vi "DataXML addNode.vi"(6 "allow repeat? (F)":bool, 7 "add_root? (F)":bool, 8 "error in (no error)":errorcluster, 9 "add tag name":string, 10 "parent node":refnum<k20>, 11 "DataXML in":refnum<class "DataXML.lvclass">) -> (0 "error out":errorcluster, 2 "new element":refnum<k20>, 3 "DataXML out":refnum<class "DataXML.lvclass">)   [LabVIEW 2018, in "DataXML.lvclass"]
uses:
  DataXML.lvclass
  DataXML.lvclass/DataXML.ctl
  <resource>/objmgr/DOMUserDefRef.rc
  <vilib>/xml/NI_XML.lvlib
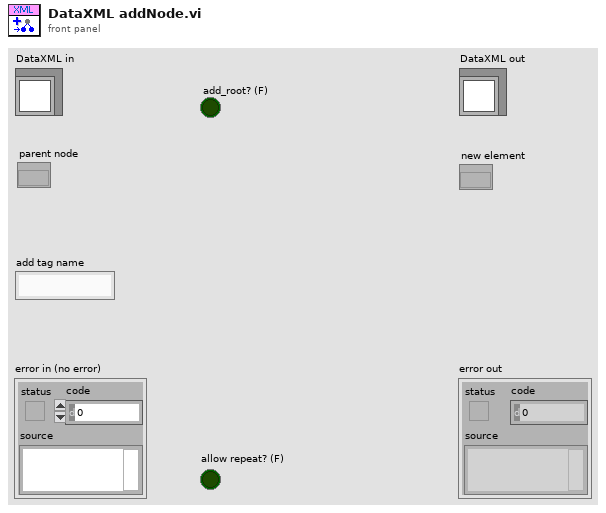
[diagram p1: front panel]
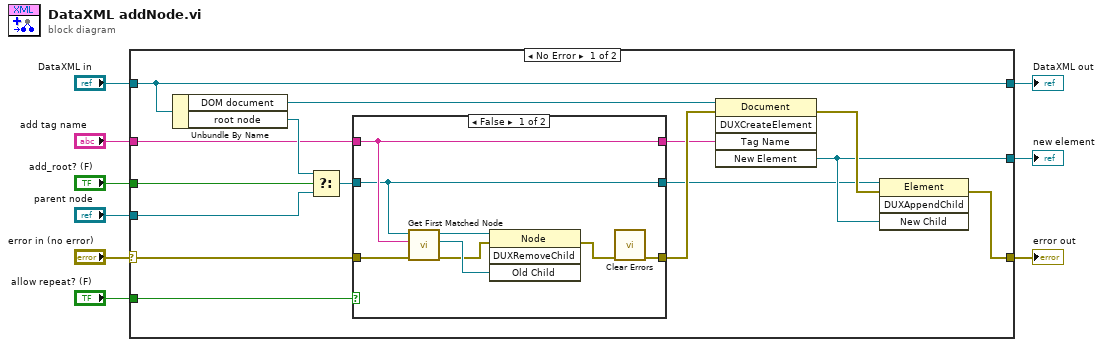
[diagram p0: block diagram]
diagram:
  n1 = case shown="No Error" "error in (no error)" {
    selector: "error in (no error)" -> [w15 w37]
    tunnel: [w18 w37] -> w8
    tunnel: [w24 w36] -> w6
    tunnel: "DataXML in" -> [w24 w36]
    tunnel: "parent node" -> [w21 _]
    tunnel: "add tag name" -> [w16 _]
    tunnel: "add_root? (F)" -> [w20 _]
    tunnel: [w17 _] -> w2
    tunnel: "allow repeat? (F)" -> [w13 _]
    frame No Error {
      n2 = Unbundle By Name(w24) -> ("DOM document"=w23:refnum<k20>, "root node"=w22:refnum<k20>)
      n3 = Select(t=w22, s=w20, f=w21) -> (s? t:f=w11:refnum<k20>)
      n4 = case shown="False" w13 {
        tunnel: w16 -> [w26 w35]
        tunnel: w15 -> [w32 w33]
        tunnel: [w27 w33] -> w14
        tunnel: [w25 w34] -> w12
        tunnel: w11 -> [w25 w34]
        tunnel: [w26 w35] -> w10
        frame False {
          n5 = call <vilib>:"Get First Matched Node.vi"("error in (no error)"=w32, "XPath expression"=w26, "node in"=w25) -> ("error out"=w29:errorcluster, "node result"=w30:refnum<k20>, "node out"=w31:refnum<k20>)  [unwired: 6 in]
          n6 = invoke class="Node" method="DUXRemoveChild"(reference=w31, error in=w29, "Old Child"=w30) -> (error out=w28:errorcluster)  [unwired: 1 in, 3 out]
          n7 = call <vilib>:"Clear Errors.vi"("error in (no error)"=w28) -> ("error out"=w27:errorcluster)  [unwired: 5 in, 1 out]
        }
        frame True {
        }
      }
      n8 = invoke class="Document" method="DUXCreateElement"(reference=w23, error in=w14, "Tag Name"=w10) -> (error out=w19:errorcluster, "New Element"=w17:refnum<k20>)  [unwired: 2 in, 3 out]
      n9 = invoke class="Element" method="DUXAppendChild"(reference=w12, error in=w19, "New Child"=w17) -> (error out=w18:errorcluster)  [unwired: 1 in, 3 out]
    }
    frame Error {
    }
  }
  "error out" <- w8
  "DataXML out" <- w6
  "new element" <- w2
